vi "Parse XML Heap.vi"(8 "error in (no error)":errorcluster, 11 "XML":string) -> (0 "error out":errorcluster, 3 "Root Element":refnum<class "Attribute.lvclass">)   [LabVIEW 2023, in "VILab.lvlib"]
uses:
  VILab.lvlib
  Classes/Attribute/Attribute.lvclass
  <vilib>/xml/Load XML String.vi
  <vilib>/xml/Close Reference(Node).vi
  <vilib>/xml/NI_XML.lvlib
  <resource>/objmgr/DOMUserDefRef.rc
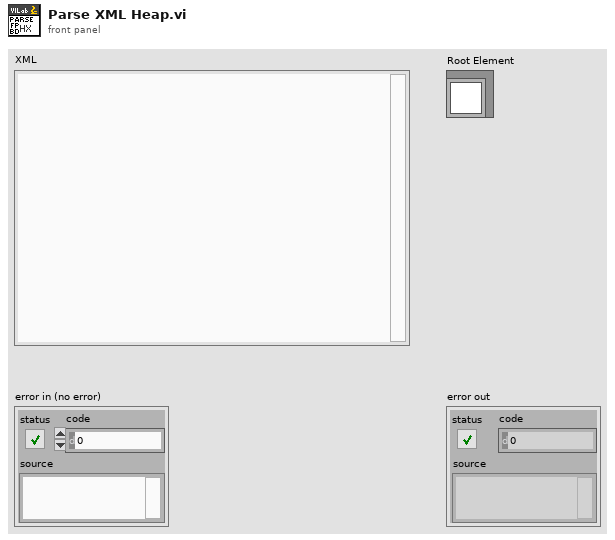
[diagram p1: front panel]
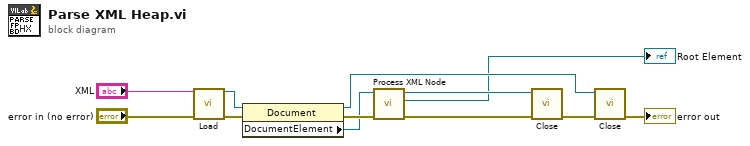
[diagram p0: block diagram]
diagram:
  n1 = call-poly <vilib>:"Load.vi"("XML string"="XML", "error in (no error)"="error in (no error)") -> ("DOM document out"=w5:refnum<k20>, "error out"=w12:errorcluster)  [unwired: 11 in, 1 out]
  n2 = property class="Document"(reference=w5, error in=w12) -> (reference out=w2:refnum<k20>, error out=w11:errorcluster, "DocumentElement"=w4:refnum<k20>)
  n3 = call "Process XML Node.vi"("error in (no error)"=w11, "node in"=w4) -> ("error out"=w9:errorcluster, "Attribute"=→"Root Element":refnum<class "Attribute.lvclass">, "node out"=w3:refnum<k20>)  [unwired: 7 in]
  n4 = call-poly <vilib>:"Close.vi"("error in (no error)"=w9, "node"=w3) -> ("error out"=w10:errorcluster)  [unwired: 7 in]
  n5 = call-poly <vilib>:"Close.vi"("error in (no error)"=w10, "node"=w2) -> ("error out"=→"error out":errorcluster)  [unwired: 7 in]
